vi "Unflatten XML Priv.vi"(0 "Tree Dict in":variant, 2 "Data Types Dict":variant, 5 "DOM Doc In":refnum<k20>, 7 "Parent Element":refnum<k20>, 9 "Parent ID":string, 11 "Error In":errorcluster) -> (4 "Tree Dict out":variant, 6 "DOM Doc Out":refnum<k20>, 8 "Parent Element":refnum<k20>, 15 "Error Out":errorcluster)   [LabVIEW 2016, in "Tree Manager.lvclass"]
uses:
  Tree Manager.lvclass
  Typedefs/Tree.ctl
  Tree Data/Tree Data.lvclass
  <vilib>/xml/Close Reference(Node).vi
  <resource>/objmgr/DOMUserDefRef.rc
  <vilib>/xml/NI_XML.lvlib
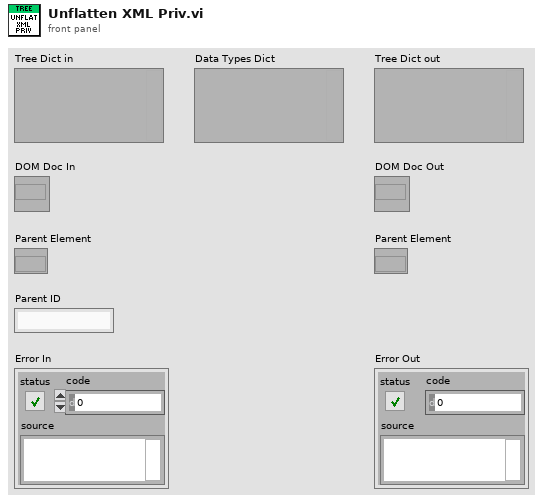
[diagram p1: front panel]
types:
  T1 = typedef "Tree Manager.lvclass/Tree.ctl" = cluster{"Unique ID":string, "Parent ID":string, "Child IDs":string[], "Data":variant, "Name":string}
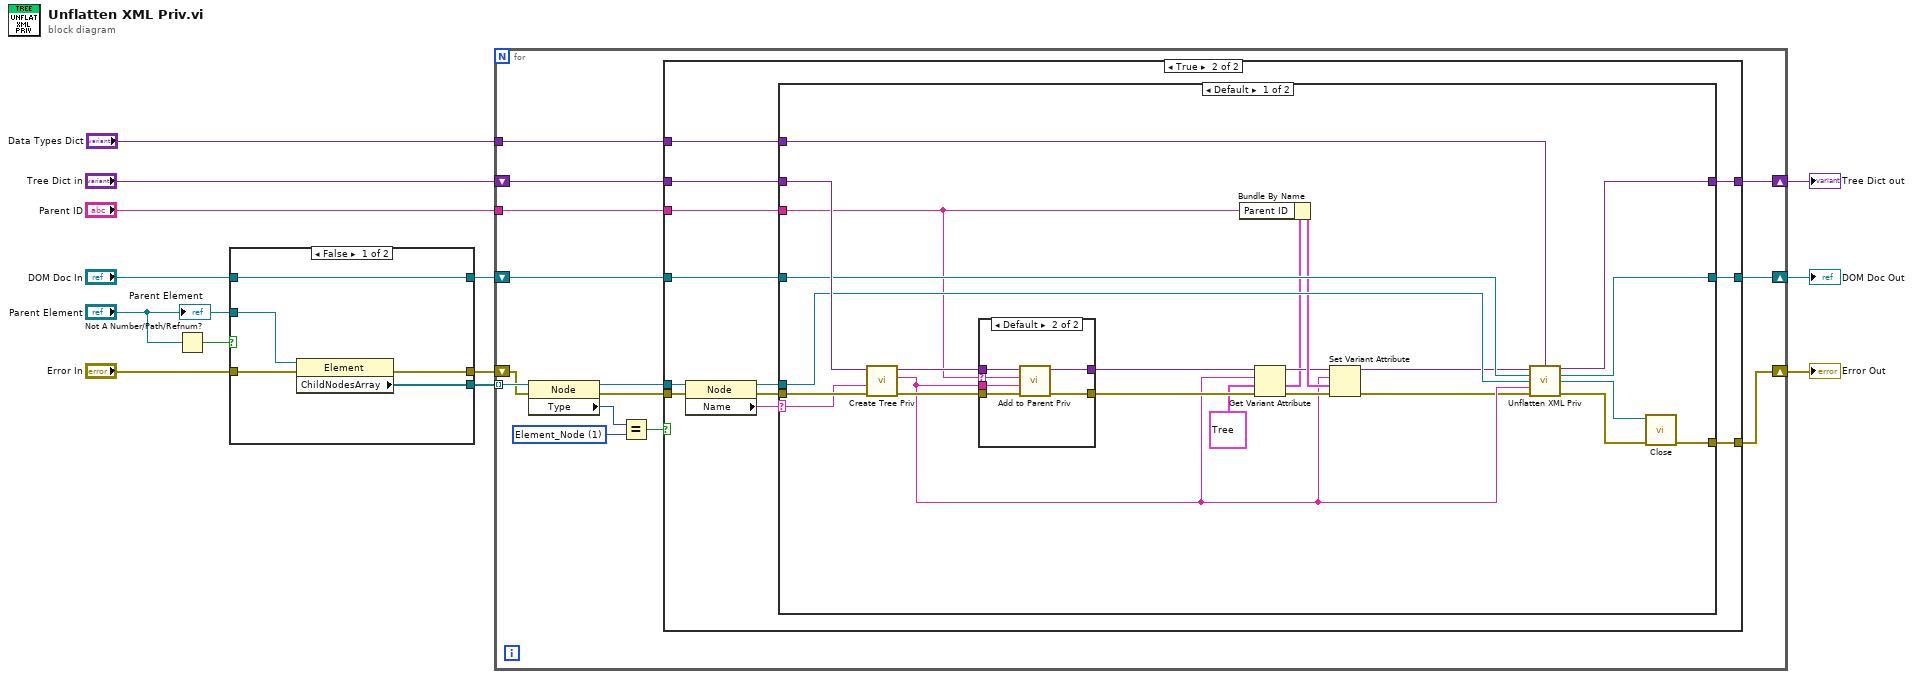
[diagram p0: block diagram]
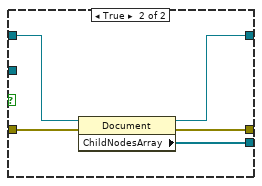
[diagram p2: hidden frame]
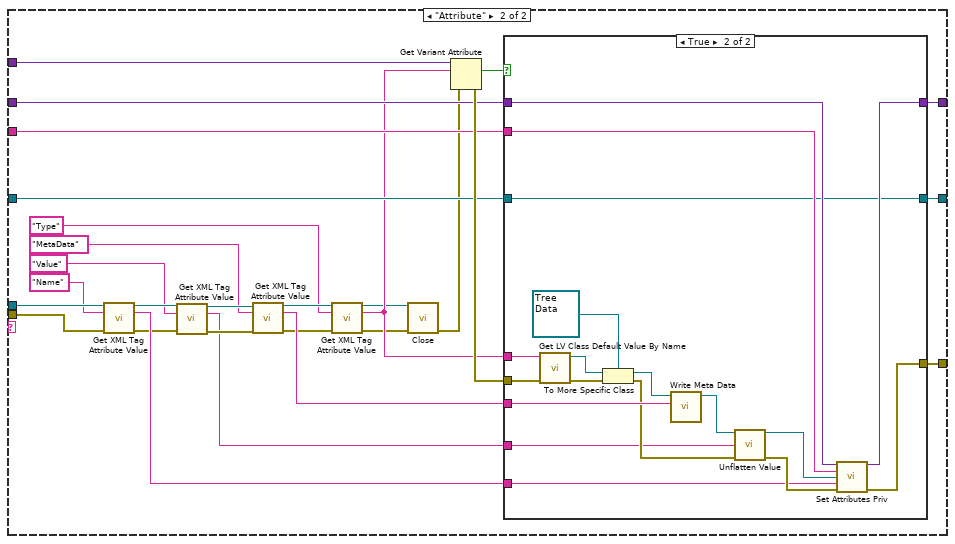
[diagram p5: hidden frame]
diagram:
  n1 = Not A Number/Path/Refnum?(number/path/refnum="Parent Element") -> (NaN/Path/Refnum?=w12:bool)
  n2 = case shown="False" w12 {
    tunnel: "DOM Doc In" -> [w18 w21]
    tunnel: [w18 w20] -> w11
    tunnel: "Parent Element" -> [w17 _]
    tunnel: "Error In" -> [w16 w23]
    tunnel: [w15 w22] -> w3
    tunnel: [w14 w19] -> w10
    frame False {
      n3 = property class="Element"(reference=w17, error in=w16) -> (error out=w15:errorcluster, "ChildNodesArray"=w14:refnum<k20>[])  [unwired: 1 out]
    }
    frame True {
      n4 = property class="Document"(reference=w21, error in=w23) -> (reference out=w20:refnum<k20>, error out=w22:errorcluster, "ChildNodesArray"=w19:refnum<k20>[])
    }
  }
  n5 = for {
    shift-right: [w34] -> w5
    shift-left: w11 -> [w35]
    tunnel: w10 -> [w30] mode=indexing
    shift-right: [w36] -> w6
    shift-left: "Tree Dict in" -> [w37]
    shift-right: [w31] -> w4
    shift-left: w3 -> [w29]
    tunnel: "Parent ID" -> [w33]
    tunnel: "Data Types Dict" -> [w32]
    w25 = 1 items=["Element_Node"=1, "Attribute_Node"=2, "Text_Node"=3, "CDATASection_Node"=4, "EntityReference_Node"=5, "Entity_Node"=6, "ProcessingInstruction_Node"=7, "Comment_Node"=8, "Document_Node"=9, "DocumentType_Node"=10, "DocumentFragment_Node"=11, "Notation_Node"=12] ("Node Type")
    n6 = property class="Node"(reference=w30, error in=w29) -> (reference out=w28:refnum<k20>, error out=w27:errorcluster, "Type"=w24:i32)
    n7 = Equal?(x=w24, y=w25) -> (x = y?=w26:bool)
    n8 = case shown="True" w26 {
      tunnel: w37 -> [w40 w50]
      tunnel: [w40 w49] -> w36
      tunnel: w35 -> [w39 w47]
      tunnel: [w39 w46] -> w34
      tunnel: w33 -> [_ w45]
      tunnel: w32 -> [_ w44]
      tunnel: [w38 w43] -> w31
      tunnel: w28 -> [_ w42]
      tunnel: w27 -> [w38 w41]
      frame False {
      }
      frame True {
        n9 = property class="Node"(reference=w42, error in=w41) -> (reference out=w48:refnum<k20>, error out=w51:errorcluster, "Name"=w52:string)
        n10 = case shown="Default" w52 {
          selector: w52 -> [w74 _]
          tunnel: w51 -> [w76 w101]
          tunnel: w50 -> [w75 w109]
          tunnel: [w71 w107] -> w49
          tunnel: w48 -> [w73 w102]
          tunnel: w47 -> [w72 w105]
          tunnel: [w70 w106] -> w46
          tunnel: w45 -> [w55 w108]
          tunnel: w44 -> [w67 w112]
          tunnel: [w64 w104] -> w43
          frame Default {
            n11 = call "Create Tree Priv.vi"("Error In"=w76, "Name"=w74, "Tree Dictionary In"=w75) -> ("Error Out"=w68:errorcluster, "Unique ID"=w57:string, "Tree Dictionary Out"=w69:variant)  [unwired: 6 in]
            n12 = case shown="Default" w55 {
              selector: w55 -> [_ w79]
              tunnel: w69 -> [w78 w84]
              tunnel: w68 -> [w77 w83]
              tunnel: [w78 w82] -> w60
              tunnel: [w77 w81] -> w59
              tunnel: w57 -> [_ w80]
              frame "" {
              }
              frame Default {
                n13 = call "Add to Parent Priv.vi"("Error In"=w83, "Unique ID"=w80, "Parent ID"=w79, "Tree Dictionary"=w84) -> ("Error Out"=w81:errorcluster, "Tree Dictionary Out"=w82:variant)  [unwired: 6 in]
              }
            }
            n14 = Get Variant Attribute(Variant=w60, name=w57, default value (empty Variant)=T1 {"Unique ID"="", "Parent ID"="", "Child IDs"=[], "Data"=variant, "Name"=""} ("output cluster"), error in=w59) -> (duplicate Variant=w61:variant, value=w56:T1, error out=w62:errorcluster)  [unwired: 1 out]
            n15 = Bundle By Name(cluster=w56, "Parent ID"=w55) -> (w63:T1)
            n16 = Set Variant Attribute(Variant=w61, name=w57, value=w63, error in=w62) -> (Variant out=w54:variant, error out=w53:errorcluster)  [unwired: 1 out]
            n17 = call "Unflatten XML Priv.vi"("Tree Dict in"=w54, "Data Types Dict"=w67, "DOM Doc In"=w72, "Parent Element"=w73, "Parent ID"=w57, "Error In"=w53) -> ("Tree Dict out"=w71:variant, "DOM Doc Out"=w70:refnum<k20>, "Parent Element"=w66:refnum<k20>, "Error Out"=w65:errorcluster)  [unwired: 6 in]
            n18 = call-poly <vilib>:"Close.vi"("error in (no error)"=w65, "node"=w66) -> ("error out"=w64:errorcluster)  [unwired: 7 in]
          }
          frame "Attribute" {
            n19 = call "Get XML Tag Attribute Value.vi"("Element In"=w102, "Name"="Name" ("Tag Name"), "error in"=w101) -> ("Element Out"=w99:refnum<k20>, "Value"=w97:string, "error out"=w96:errorcluster)  [unwired: 10 in]
            n20 = call "Get XML Tag Attribute Value.vi"("Element In"=w99, "Name"="Value" ("Tag Name"), "error in"=w96) -> ("Element Out"=w98:refnum<k20>, "Value"=w93:string, "error out"=w94:errorcluster)  [unwired: 10 in]
            n21 = call "Get XML Tag Attribute Value.vi"("Element In"=w98, "Name"="MetaData" ("Tag Name"), "error in"=w94) -> ("Element Out"=w90:refnum<k20>, "Value"=w91:string, "error out"=w89:errorcluster)  [unwired: 10 in]
            n22 = call "Get XML Tag Attribute Value.vi"("Element In"=w90, "Name"="Type" ("Tag Name"), "error in"=w89) -> ("Element Out"=w85:refnum<k20>, "Value"=w87:string, "error out"=w86:errorcluster)  [unwired: 10 in]
            n23 = call-poly <vilib>:"Close.vi"("error in (no error)"=w86, "node"=w85) -> ("error out"=w103:errorcluster)  [unwired: 7 in]
            n24 = Get Variant Attribute(Variant=w112, name=w87, error in=w103) -> (found=w111:bool, error out=w110:errorcluster)  [unwired: 1 in, 2 out]
            n25 = case shown="True" w111 {
              tunnel: w87 -> [_ w133]
              tunnel: w110 -> [w113 w132]
              tunnel: w91 -> [_ w127]
              tunnel: w93 -> [_ w124]
              tunnel: w109 -> [w115 w123]
              tunnel: w108 -> [_ w121]
              tunnel: [w115 w120] -> w107
              tunnel: w97 -> [_ w118]
              tunnel: [w114 w117] -> w106
              tunnel: w105 -> [w114 w117]
              tunnel: [w113 w116] -> w104
              frame False {
              }
              frame True {
                n26 = call <vilib>:"Get LV Class Default Value By Name.vi"("error in (no error)"=w132, "class name"=w133) -> ("error out"=w131:errorcluster, "object"=w130:refnum<class>)  [unwired: 8 in]
                n27 = To More Specific Class(target class=refnum<class "Tree Data.lvclass"> refnum ("Tree Data.lvclass"), reference=w130, error in=w131) -> (specific class reference=w128:refnum<class "Tree Data.lvclass">, error out=w125:errorcluster)
                n28 = call "Write Meta Data.vi"("Meta Data"=w127, "Tree Data In"=w128) -> ("Tree Data Out"=w126:refnum<class "Tree Data.lvclass">)  [unwired: 9 in]
                n29 = call-dynamic "Unflatten Value.vi"("Tree Data In"=w126, "Value"=w124, "Error In"=w125) -> ("Tree Data Out"=w119:refnum<class "Tree Data.lvclass">, "Error Out"=w122:errorcluster)  [unwired: 11 in]
                n30 = call "Set Attributes Priv.vi"("Tree Dictionary Out"=w123, "Unique ID"=w121, "Data"=w119, "Name"=w118, "error in"=w122) -> ("Tree Dictionary Out"=w120:variant, "error out"=w116:errorcluster)  [unwired: 8 in, 1 out]
              }
            }
          }
        }
      }
    }
  }
  "Error Out" <- w4
  "Tree Dict out" <- w6
  "DOM Doc Out" <- w5
  "Parent Element" <- "Parent Element"
